vi "SetChangeTaskSampleTrigger.vi"(0 "controller in":refnum<k24>, 5 "signal":u32(ring)=17 items=["ActiveFixtureOffset"=106, "ActiveMoveValid"=435, "AxesSlowdownReason"=448, "CannedFunctionID"=240, "CoordinatedAccelerationCommand"=64, "CoordinatedAccelerationRate"=132, "CoordinatedAccelerationTime"=134, "CoordinatedArcEndAngle"=59, "CoordinatedArcRadius"=60, "CoordinatedArcRadiusError"=61, "CoordinatedArcRadiusReciprocal"=363, "CoordinatedArcStartAngle"=58, "CoordinatedDecelerationRate"=133, "CoordinatedDecelerationTime"=135, "CoordinatedFlags"=45, "CoordinatedGalvoLaserOutput"=169, "CoordinatedMotionRate"=184, "CoordinatedPercentDone"=66, "CoordinatedPositionCommand"=62, "CoordinatedPositionCommandBackwardsDiff"=67, "CoordinatedSpeedCommand"=63, "CoordinatedSpeedTarget"=124, "CoordinatedSpeedTargetActual"=104, "CoordinatedTaskCommand"=185, "CoordinatedTimeScale"=370, "CoordinatedTimeScaleDerivative"=371, "CoordinatedTotalDistance"=65, "CoordinateSystem1I"=118, "CoordinateSystem1J"=119, "CoordinateSystem1K"=120, "CoordinateSystem1Plane"=121, "CriticalSectionActive"=440, "DependentCoordinatedSpeedTarget"=125, "DependentCoordinatedSpeedTargetActual"=105, "EnableAlignmentAxes"=159, "EnableState"=224, "ExecutionMode"=151, "FiberMoveCount"=195, "FiberPower"=273, "FiberPowerOptimal"=274, "FiberPowerSampleCount"=275, "FiberSearchResult"=276, "IFOVAttemptCode"=394, "IFOVCenterPointH"=390, "IFOVCenterPointV"=391, "IFOVCoordinatedAccelerationCommand"=399, "IFOVCoordinatedPositionCommand"=385, "IFOVCoordinatedSpeedCommand"=386, "IFOVFOVDimensionH"=402, "IFOVFOVDimensionV"=403, "IFOVFOVPositionH"=400, "IFOVFOVPositionV"=401, "IFOVGenerationFrameCounter"=382, "IFOVGenerationFrameIndex"=395, "IFOVGenerationTimeModified"=384, "IFOVGenerationTimeOriginal"=383, "IFOVIdealVelocity"=397, "IFOVMaximumVelocity"=396, "IFOVSpeedScale"=380, "IFOVSpeedScaleAverage"=381, "IFOVTrajectoryCount"=392, "IFOVTrajectoryIndex"=393, "ImmediateCommandErrorCode"=329, "ImmediateCommandErrorLocation"=330, "ImmediateState"=155, "LookaheadMovesExamined"=278, "MFO"=123, "MotionBufferElements"=427, "MotionBufferIndex"=432, "MotionBufferIndexLookahead"=433, "MotionBufferMoves"=428, "MotionBufferProcessingBlocked"=434, "MotionBufferRetraceElements"=431, "MotionBufferRetraceMoves"=430, "MotionEngineStage"=367, "MotionLineNumber"=429, "ProfileControlMask"=324, "ProgramLineNumber"=17, "ProgramLineNumberInternal"=322, "ProgramPersistent"=154, "ProgramVariable"=75, "QueueLineCapacity"=326, "QueueLineCount"=325, "QueueStatus"=162, "SchedulerProgramLoopRuns"=438, "SchedulerTaskBlocked"=439, "SchedulerTaskHolds"=437, "Spindle0SpeedTarget"=112, "Spindle1SpeedTarget"=113, "Spindle2SpeedTarget"=114, "Spindle3SpeedTarget"=115, "TaskDoubleVariable"=248, "TaskErrorCode"=79, "TaskErrorLocation"=152, "TaskExecutionLines"=436, "TaskExecutionLinesMaximum"=452, "TaskExecutionTime"=450, "TaskExecutionTimeMaximum"=451, "TaskInfoVariable"=249, "TaskInternalDebug"=398, "TaskMode"=137, "TaskParameter"=77, "TaskReturnVariable"=271, "TaskState"=146, "TaskStateInternal"=147, "TaskStatus0"=108, "TaskStatus1"=109, "TaskStatus2"=110, "TaskWarningCode"=80, "TaskWarningLocation"=153, "ToolNumberActive"=122, "WaitCommandDuration"=103], 7 "task":i32, 9 "optional":i32, 11 "error in (no error)":errorcluster, 12 "trigger":i32(ring)=1 items=["OnAnyChange"=1, "OnIncrease"=2, "OnDecrease"=3]) -> (4 "controller out":refnum<k24>, 15 "error out":errorcluster)   [LabVIEW 2020, in "Aerotech.lvlib"]
uses:
  Aerotech.lvlib
  C:/Users/HEP/Documents/GitHub/UCSB-Gantry-HEP/Drivers/Aerotech A3200/Bin/Aerotech.A3200.LabVIEW.dll
  UCSB-Gantry-HEP/Drivers/Aerotech A3200/Bin/Aerotech.A3200.LabVIEW.dll
  C:/Program Files (x86)/Aerotech/A3200/LabVIEW/2010/Bin/Aerotech.A3200.dll
  Program Files (x86)/Aerotech/A3200/LabVIEW/2010/Bin/Aerotech.A3200.dll
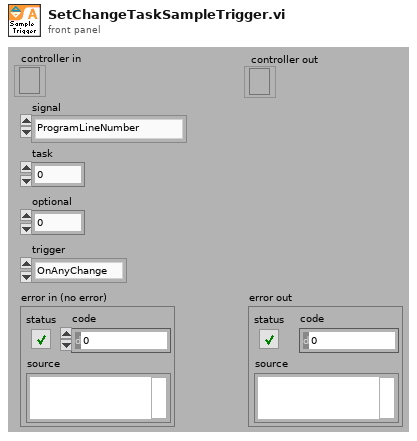
[diagram p1: front panel]
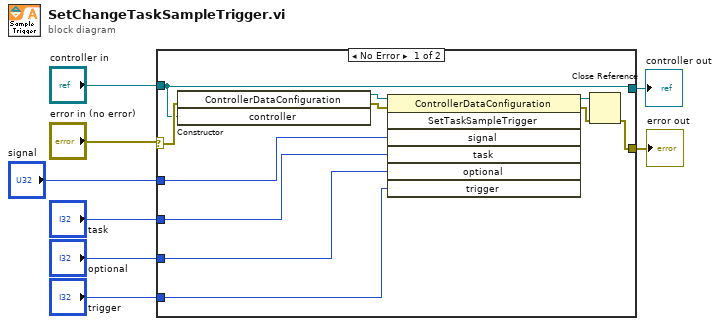
[diagram p0: block diagram]
diagram:
  n1 = case shown="No Error" "error in (no error)" {
    selector: "error in (no error)" -> [w19 w21]
    tunnel: "controller in" -> [w14 w20]
    tunnel: [w11 w21] -> w5
    tunnel: [w14 w20] -> w6
    tunnel: "optional" -> [w15 _]
    tunnel: "trigger" -> [w16 _]
    tunnel: "task" -> [w10 _]
    tunnel: "signal" -> [w9 _]
    frame No Error {
      n2 = constructor class="ControllerDataConfiguration"(error in=w19, "controller"=w14) -> (reference out=w18:refnum<k24>, error out=w17:errorcluster)  [unwired: 2 in, 2 out]
      n3 = invoke class="ControllerDataConfiguration" method="SetTaskSampleTrigger"(reference=w18, error in=w17, "signal"=w9, "task"=w10, "optional"=w15, "trigger"=w16) -> (reference out=w12:refnum<k24>, error out=w13:errorcluster)  [unwired: 1 in, 5 out]
      n4 = Close Reference(reference=w12, error in (no error)=w13) -> (error out=w11:errorcluster)
    }
    frame Error {
    }
  }
  "controller out" <- w6
  "error out" <- w5
